vi "List to List Info.vi"(8 "error in (no error)":errorcluster, 10 "List String":string, 11 "FTP in":refnum<class "FTP.lvclass">) -> (0 "error out":errorcluster, 1 "invalid data":bool, 2 "Dir-File Info":T1, 3 "FTP out":refnum<class "FTP.lvclass">)   [LabVIEW 2020, in "FTP.lvlib" / "FTP.lvclass"]
uses:
  FTP.lvclass
  controls/Dir-File Info.ctl
  controls/Dir-File Type.ctl
  FTP.lvclass/FTP.ctl
  <vilib>/Utility/error.llb/whitespace.ctl
  <vilib>/Utility/miscctls.llb/LVDateTimeRec.ctl
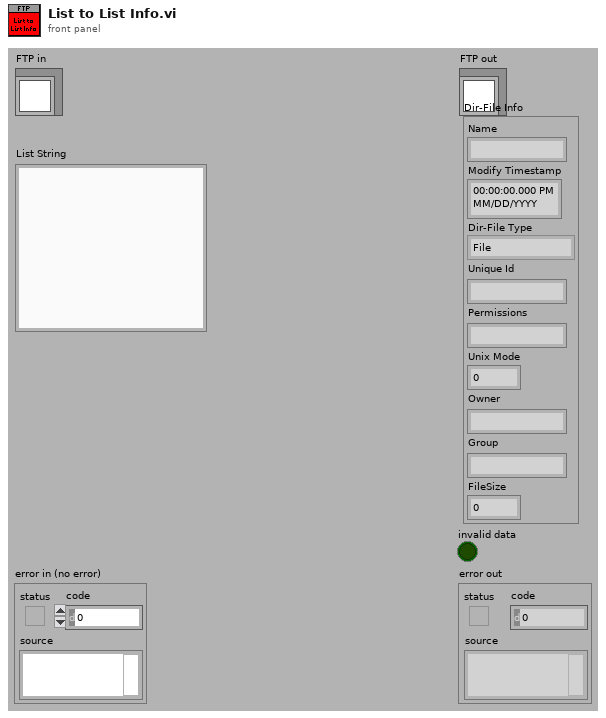
[diagram p1: front panel]
types:
  T1 = typedef "FTP.lvlib/FTP.lvclass/Dir-File Info.ctl" = cluster{"Name":string, "Modify Timestamp":timestamp, "Dir-File Type":T2, "Unique Id":string, "Permissions":string, "Unix Mode":u16, "Owner":string, "Group":string, "FileSize":i64}
  T2 = typedef "FTP.lvlib/FTP.lvclass/Dir-File Type.ctl" = enum16{"File", "Listed Directory", "Parent Directory", "Directory", "Unknown"}
  T3 = typedef "LVDateTimeRec.ctl" = cluster{"fractional second":dbl, "second":i32, "minute":i32, "hour":i32, "day of month":i32, "month":i32, "year":i32, "day of week":i32, "day of year":i32, "DST":i32}
  T4 = typedef "whitespace.ctl" = u16
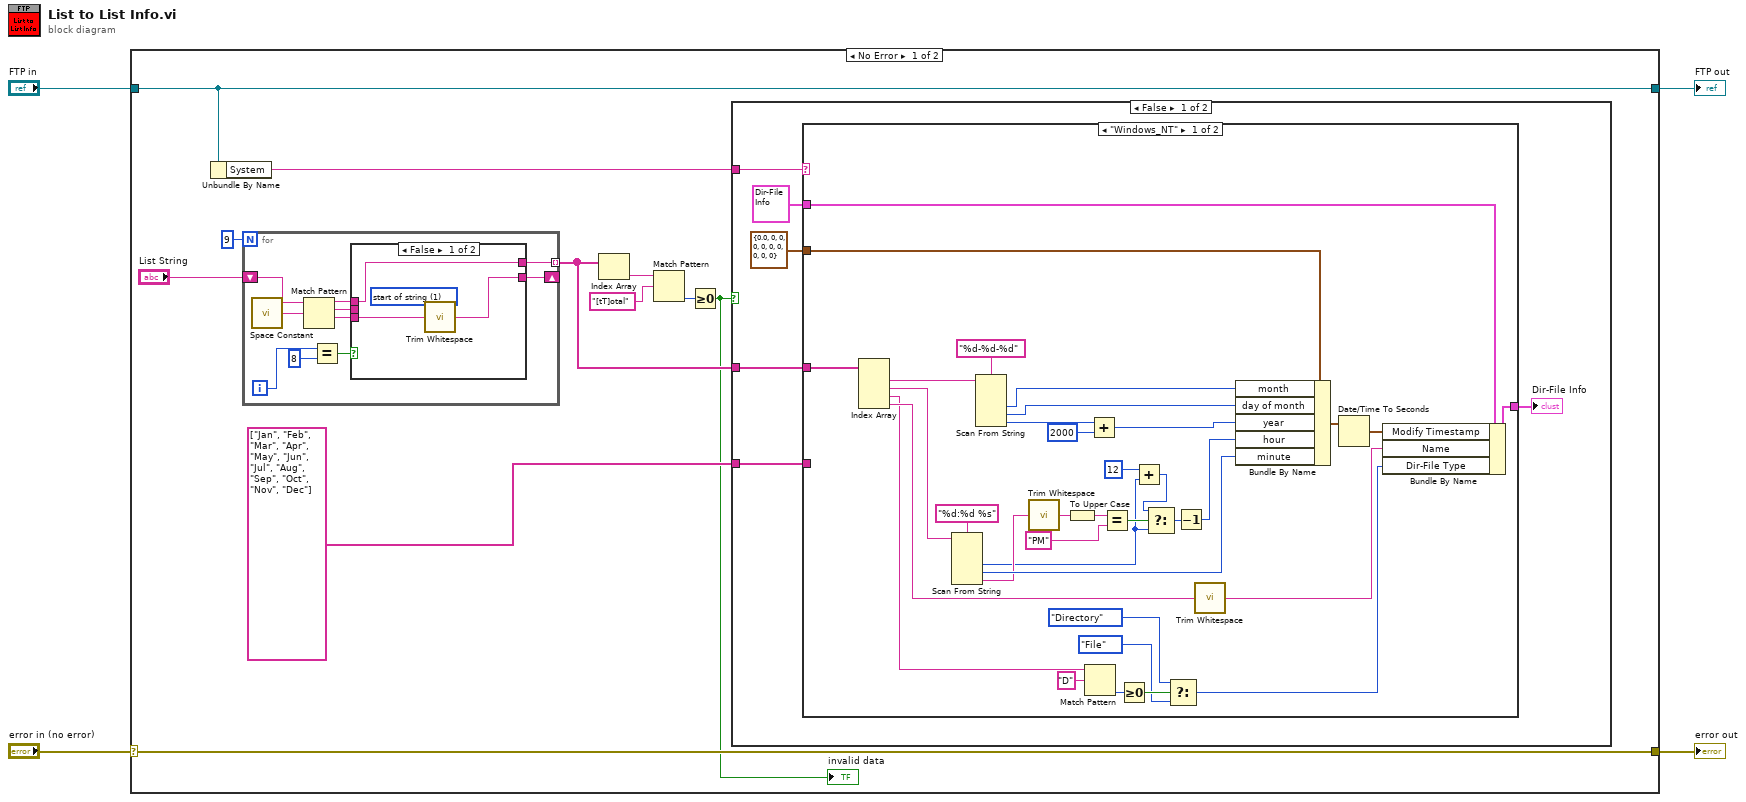
[diagram p0: block diagram]
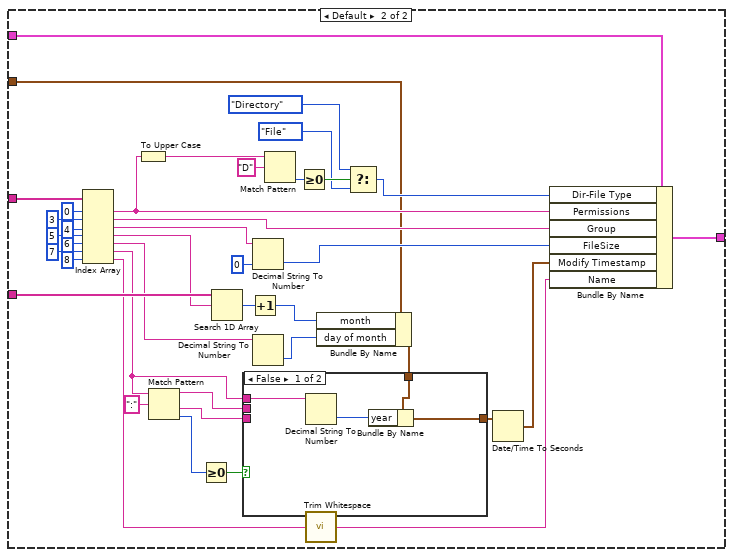
[diagram p2: hidden frame]
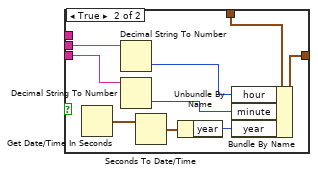
[diagram p3: hidden frame]
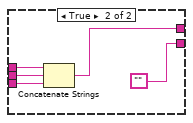
[diagram p5: hidden frame]
diagram:
  n1 = case shown="No Error" "error in (no error)" {
    selector: "error in (no error)" -> [w15 w130]
    tunnel: [w15 w130] -> w3
    tunnel: [w6 w129] -> w1
    tunnel: "FTP in" -> [w6 w129]
    frame No Error {
      n2 = Unbundle By Name(w6) -> ("System"=w5:string)
      n3 = for {
        N: 9 -> [_]
        shift-right: [w117] -> _
        shift-left: "List String" -> [w119]
        tunnel: [w111] -> w11 mode=indexing
        i -> [w114]
        n4 = call <vilib>:"Space Constant.vi"() -> ("String"=w116:string)
        n5 = Match Pattern(string=w119, regular expression=w116) -> (before substring=w112:string, match substring=w110:string, after substring=w118:string)  [unwired: 1 in, 1 out]
        n6 = Equal?(x=w114, y=8) -> (x = y?=w115:bool)
        n7 = case shown="False" w115 {
          tunnel: w118 -> [w122 w125]
          tunnel: [w121 ""] -> w117
          tunnel: w112 -> [w120 w127]
          tunnel: [w120 w124] -> w111
          tunnel: w110 -> [_ w126]
          frame False {
            w123 = T4 1 items=["both", "start of string", "end of string"] ("location (both)")
            n8 = call <vilib>:"Trim Whitespace.vi"("string"=w122, "location (both)"=w123) -> ("trimmed string"=w121:string)
          }
          frame True {
            n9 = Concatenate Strings(w127, w126, w125) -> (w124:string)
          }
        }
      }
      n10 = Index Array(array=w11) -> (element=w10:string)  [unwired: 1 in]
      n11 = Match Pattern(string=w10, regular expression="[tT]otal") -> (offset past match=w8:i32)  [unwired: 1 in, 3 out]
      n12 = Greater Or Equal To 0?(x=w8) -> (x >= 0?=w7:bool)
      "invalid data" <- w7
      n13 = case shown="False" w7 {
        tunnel: string[] ["Jan", "Feb", "Mar", "Apr", "May", "Jun", "Jul", "Aug", "Sep", "Oct", "Nov", "Dec"] -> [w21 _]
        tunnel: w11 -> [w19 _]
        tunnel: w5 -> [w18 _]
        frame False {
          n14 = case shown="\"Windows_NT\"" w18 {
            tunnel: w21 -> [_ w96]
            tunnel: [w45 w89] -> w20
            tunnel: w19 -> [w55 w59]
            tunnel: T3 {"fractional second"=0.0, "second"=0, "minute"=0, "hour"=0, "day of month"=0, "month"=0, "year"=0, "day of week"=0, "day of year"=0, "DST"=0} ("date time rec") -> [w54 w58]
            tunnel: T1 {"Name"="", "Modify Timestamp"=timestamp(0 s since 1904-01-01), "Dir-File Type"=enum."File", "Unique Id"="", "Permissions"="", "Unix Mode"=0, "Owner"="", "Group"="", "FileSize"=0} ("Dir-File Info") -> [w56 w57]
            frame "Windows_NT" {
              n15 = Index Array(array=w55) -> (element #1=w53:string, element #2=w48:string, element #3=w24:string, element #4=w30:string)  [unwired: 4 in]
              n16 = Scan From String(format string="%d:%d %s", input string=w48) -> (output 1=w34:i32, output 2=w46:i32, output 3=w40:string)  [unwired: 5 in, 3 out]
              n17 = Scan From String(format string="%d-%d-%d", input string=w53) -> (output 1=w51:i32, output 2=w50:i32, output 3=w49:i32)  [unwired: 5 in, 3 out]
              n18 = call <vilib>:"Trim Whitespace.vi"("string"=w40) -> ("trimmed string"=w39:string)  [unwired: 1 in]
              n19 = To Upper Case(1:w39) -> (0:w37:string)
              n20 = Match Pattern(string=w24, regular expression="D") -> (offset past match=w28:i32)  [unwired: 1 in, 3 out]
              n21 = Add(x=w49, y=2000) -> (x+y=w42:i32)
              n22 = Equal?(x=w37, y="PM") -> (x = y?=w36:bool)
              n23 = Greater Or Equal To 0?(x=w28) -> (x >= 0?=w27:bool)
              n24 = Add(x=12, y=w34) -> (x+y=w35:i32)
              n25 = Select(t=w35, s=w36, f=w34) -> (s? t:f=w32:i32)
              n26 = Select(t=Dir-File_Type."Directory" ("Dir-File Type"), s=w27, f=Dir-File_Type."File" ("Dir-File Type")) -> (s? t:f=w23:T2)
              n27 = Decrement(x=w32) -> (x-1=w31:i32)
              n28 = call <vilib>:"Trim Whitespace.vi"("string"=w30) -> ("trimmed string"=w22:string)  [unwired: 1 in]
              n29 = Bundle By Name(cluster=w54, "month"=w51, "day of month"=w50, "year"=w42, "hour"=w31, "minute"=w46) -> (w44:T3)
              n30 = Date/Time To Seconds(2:w44) -> (0:w43:timestamp)  [unwired: 1 in]
              n31 = Bundle By Name(cluster=w56, "Modify Timestamp"=w43, "Name"=w22, "Dir-File Type"=w23) -> (w45:T1)
            }
            frame Default {
              n32 = Index Array(array=w59, index #1=0 ("index"), index #2=3 ("index"), index #3=4 ("index"), index #4=5 ("index"), index #5=6 ("index"), index #6=7 ("index"), index #7=8 ("index")) -> (element #1=w79:string, element #2=w91:string, element #3=w88:string, element #4=w63:string, element #5=w85:string, element #6=w71:string, element #7=w81:string)
              n33 = To Upper Case(1:w79) -> (0:w77:string)
              n34 = Match Pattern(string=w71, regular expression=":") -> (before substring=w65:string, after substring=w64:string, offset past match=w69:i32)  [unwired: 1 in, 1 out]
              n35 = Greater Or Equal To 0?(x=w69) -> (x >= 0?=w66:bool)
              n36 = Search 1D Array(1D array=w96, element=w63) -> (index of element=w62:i32)  [unwired: 1 in]
              n37 = Increment(x=w62) -> (x+1=w61:i32)
              n38 = Decimal String To Number(string=w88, default (0L)=i64 0 ("default (0 I32)")) -> (number=w87:i64)  [unwired: 1 in, 1 out]
              n39 = Decimal String To Number(string=w85) -> (number=w60:i32)  [unwired: 2 in, 1 out]
              n40 = Match Pattern(string=w77, regular expression="D") -> (offset past match=w76:i32)  [unwired: 1 in, 3 out]
              n41 = Greater Or Equal To 0?(x=w76) -> (x >= 0?=w75:bool)
              n42 = call <vilib>:"Trim Whitespace.vi"("string"=w81) -> ("trimmed string"=w80:string)  [unwired: 1 in]
              n43 = Bundle By Name(cluster=w58, "month"=w61, "day of month"=w60) -> (w68:T3)
              n44 = case shown="False" w66 {
                tunnel: w71 -> [w100 _]
                tunnel: w68 -> [w99 w105]
                tunnel: [w98 w106] -> w67
                tunnel: w65 -> [_ w103]
                tunnel: w64 -> [_ w102]
                frame False {
                  n45 = Decimal String To Number(string=w100) -> (number=w97:i32)  [unwired: 2 in, 1 out]
                  n46 = Bundle By Name(cluster=w99, "year"=w97) -> (w98:T3)
                }
                frame True {
                  n47 = Get Date/Time In Seconds() -> (seconds since 1Jan1904=w109:timestamp)
                  n48 = Decimal String To Number(string=w103) -> (number=w104:i32)  [unwired: 2 in, 1 out]
                  n49 = Decimal String To Number(string=w102) -> (number=w101:i32)  [unwired: 2 in, 1 out]
                  n50 = Seconds To Date/Time(time stamp (now)=w109) -> (date time rec=w108:T3)  [unwired: 1 in]
                  n51 = Unbundle By Name(w108) -> ("year"=w107:i32)
                  n52 = Bundle By Name(cluster=w105, "hour"=w104, "minute"=w101, "year"=w107) -> (w106:T3)
                }
              }
              n53 = Select(t=Dir-File_Type."Directory" ("Dir-File Type"), s=w75, f=Dir-File_Type."File" ("Dir-File Type")) -> (s? t:f=w72:T2)
              n54 = Date/Time To Seconds(2:w67) -> (0:w90:timestamp)  [unwired: 1 in]
              n55 = Bundle By Name(cluster=w57, "Dir-File Type"=w72, "Permissions"=w79, "Group"=w91, "FileSize"=w87, "Modify Timestamp"=w90, "Name"=w80) -> (w89:T1)
            }
          }
          "Dir-File Info" <- w20
        }
        frame True {
        }
      }
    }
    frame Error {
    }
  }
  "error out" <- w3
  "FTP out" <- w1
